vi "Rx Inline Wait.vi"(8 "error in (no error)":errorcluster, 11 "Plugin in":refnum<class "Plugin.lvclass">) -> (0 "error out":errorcluster, 3 "Plugin out":refnum<class "Plugin.lvclass">)   [LabVIEW 2019, in "DSF Core.lvlib" / "Plugin.lvclass"]
uses:
  Plugin.lvclass
  Plugin.lvclass/Plugin.ctl
  Transfer Group/Transfer Group.lvclass/Transfer Group.ctl
  Timing/Timing.lvclass/Timing.ctl
  Transfer Group/Retrieve from FIFO.vi
  Transfer Group/Get Iteration and Late Count.vi
  Transfer Group/Increment Iteration.vi
  Transfer Group/Is Late.vi
  Transfer Group/Read Return FIFO.vi
  Transfer Group/Errors.vi
  Transfer Group/Invalid Iteration Error.vi
  Timing/Get Iteration.vi
  Timing/Increment Iteration.vi
  Transfer Group/Increment Late Count.vi
  Transfer Group/Return Timeout Error.vi
  VIs/Constants/Constants.vi
  VIs/Constants/Engine Library Name.vi
  <vilib>/NI/Memory Manager/VIs/New Error Cluster.vi
  <vilib>/NI/Memory Manager/VIs/New Error Cluster (512B).vi
  <vilib>/NI/Memory Manager/VIs/Set Error Status.vi
  <vilib>/NI/Memory Manager/VIs/Set Error Code.vi
  <vilib>/NI/Memory Manager/VIs/Set Error Source.vi
  <vilib>/NI/Memory Manager/VIs/Write String to Source.vi
  <vilib>/NI/Memory Manager/VIs/Write Numeric to Source.vi
  <vilib>/NI/Memory Manager/VIs/Write Numeric Scalar to Source (Base10 U64).vi
  Transfer Group/Transfer Group Error Info.vi
  <vilib>/NI/Memory Manager/VIs/Write Numeric Scalar to Source (Base10 I32).vi
  VIs/Constants/Base Error Code.vi
  Transfer Group/Transfer Group Error Offset.vi
  Transfer Group/Transfer Group.lvclass
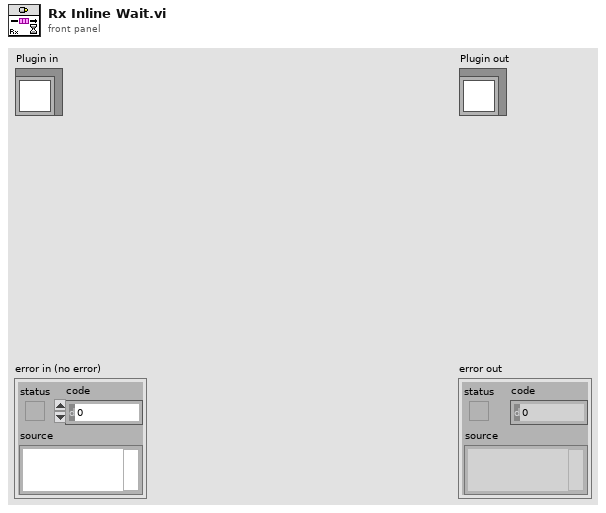
[diagram p1: front panel]
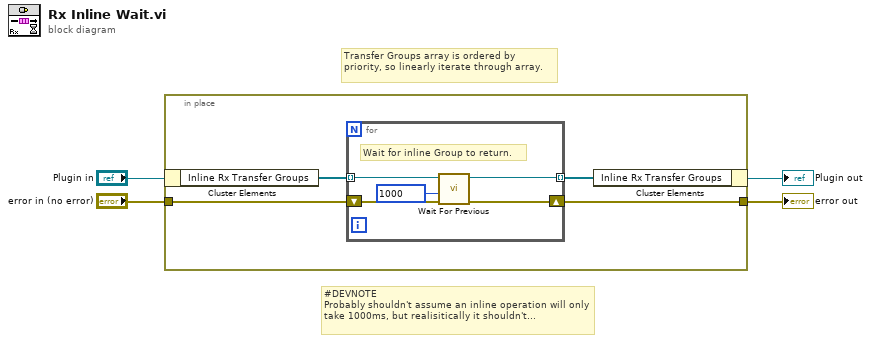
[diagram p0: block diagram]
diagram:
  # "#DEVNOTE\nProbably shouldn't assume an inline operation will only take 1000ms, but realisitically it shouldn't..."
  # "Transfer Groups array is ordered by priority, so linearly iterate through array."
  n1 = in-place {
    in-place-border: "error in (no error)" -> [w8]
    in-place-border: [w7] -> w4
    n2 = in-place-cluster #1("Plugin in") -> ("Inline Rx Transfer Groups"=w6:refnum<class "Transfer Group.lvclass">[])
    n3 = for {
      tunnel: w6 -> [w12] mode=indexing
      shift-right: [w9] -> w7
      shift-left: w8 -> [w11]
      tunnel: [w10] -> w5 mode=indexing
      # "Wait for inline Group to return."
      n4 = call "Wait For Previous.vi"("error in (no error)"=w11, "timeout in ms (0)"=1000, "Transfer Group in"=w12) -> ("error out"=w9:errorcluster, "Transfer Group out"=w10:refnum<class "Transfer Group.lvclass">)  [unwired: 5 in, 2 out]
    }
    n5 = in-place-cluster #1("Inline Rx Transfer Groups"=w5) -> (→"Plugin out":refnum<class "Plugin.lvclass">)
  }
  "error out" <- w4
